vi "messagerVI.vi"(9 "msg data in":dbl[](array[numeric]), 10 "data to change in":dbl[](array[numeric]), 11 "T=Set, F=Act":bool) -> (1 "msg data out":dbl[](array[numeric]), 2 "data to change out":dbl[](array[numeric]))   [LabVIEW 2014]
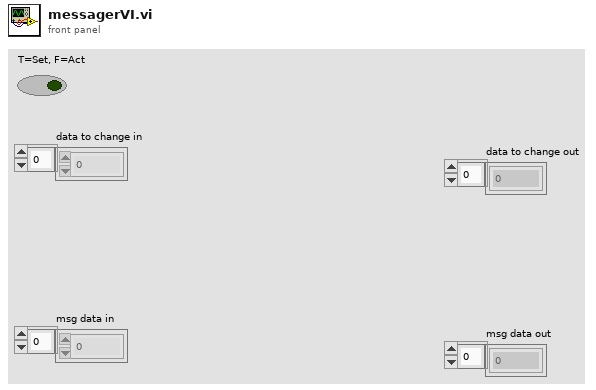
[diagram p1: front panel]
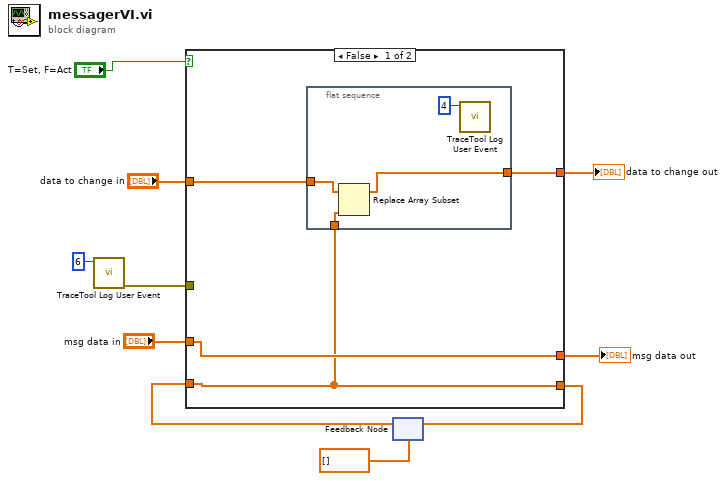
[diagram p0: block diagram]
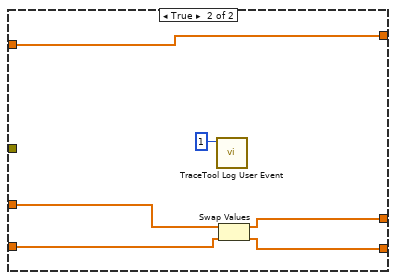
[diagram p2: hidden frame]
diagram:
  n1 = call <vilib>:"TraceTool Log User Event.vi"("Event ID (0-255)"=u32 6) -> ("error out"=w1:errorcluster)  [unwired: 10 in]
  n2 = feedback #1(dbl[] [] ("msg data in")) -> (w5:dbl[])
  n3 = case shown="False" "T=Set, F=Act" {
    tunnel: [w12 w24] -> w8
    tunnel: "data to change in" -> [w13 w24]
    tunnel: [w11 w21] -> w6
    tunnel: w5 -> [w11 w22]
    tunnel: "msg data in" -> [w14 w23]
    tunnel: [w14 w20] -> w3
    tunnel: w1 -> [_ _]
    frame False {
      n4 = flat-sequence {
        tunnel: w13 -> [w18]
        tunnel: [w17] -> w12
        tunnel: w11 -> [w16]
        frame #0 {
          n5 = Replace Array Subset(array=w18, new element=w16) -> (w17:dbl[])  [unwired: 1 in]
          n6 = call <vilib>:"TraceTool Log User Event.vi"("Event ID (0-255)"=u32 4) -> ()  [unwired: 10 in, 1 out]
        }
      }
    }
    frame True {
      n7 = call <vilib>:"TraceTool Log User Event.vi"("Event ID (0-255)"=u32 1) -> ()  [unwired: 10 in, 1 out]
      n8 = Swap Values(12:w23, 14:w22) -> (1:w20:dbl[], 3:w21:dbl[])  [unwired: 1 in]
    }
  }
  "data to change out" <- w8
  "msg data out" <- w3
  n9 = feedback-in #1(w6) -> ()
